vi "Buid Map Typenames.vi"(8 "error in (no error)":errorcluster, 9 "Message Name":string, 10 "Map Name":string) -> (0 "error out":errorcluster, 2 "Map Typenames":T1)   [LabVIEW 2020, in "LV-Protoc.lvlib" / "LV-Protoc.lvclass"]
uses:
  LV-Protoc.lvclass
  Map Typenames.ctl
  LV-Protoc.lvlib
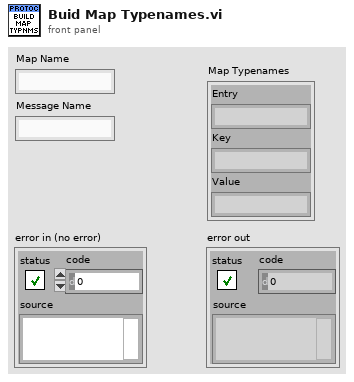
[diagram p1: front panel]
types:
  T1 = typedef "LV-Protoc.lvlib/Map Typenames.ctl" = cluster{"Entry":string, "Key":string, "Value":string}
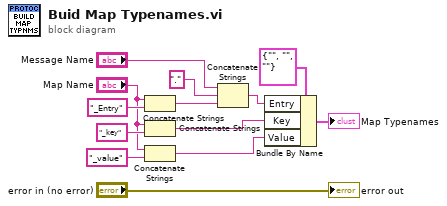
[diagram p0: block diagram]
diagram:
  n1 = Concatenate Strings("Map Name", "_Entry" ("string")) -> (w9:string)
  n2 = Concatenate Strings("Map Name", "_key" ("string")) -> (w8:string)
  n3 = Concatenate Strings("Map Name", "_value" ("string")) -> (w7:string)
  n4 = Concatenate Strings("Message Name", "." ("string"), w9) -> (w3:string)
  n5 = Bundle By Name(cluster=T1 {"Entry"="", "Key"="", "Value"=""} ("Map Typenames"), "Entry"=w3, "Key"=w8, "Value"=w7) -> (→"Map Typenames":T1)
  "error out" <- "error in (no error)"
